vi "GenCMSMismatchFile.vi"() -> ()   [LabVIEW 2016]
uses:
  CMSMismatch.ctl
  <vilib>/NI/GXML/GXML.lvlib
panel:
  in  "Save Path":path
  in  "CableMotorSensorMismatch":T1={"TotalCount"={"CableCount"=0, "MotorCount"=0, "SensorCount"=0}, "Matches"=[{"CableID"=4, "MotorID"=8, "SensorID"=8}, {"CableID"=1, "MotorID"=6, "SensorID"=8}, {"CableID"=2, "MotorID"=5, "SensorID"=5}, {"CableID"=3, "MotorID"=7, "SensorID"=4}, {"CableID"=4, "MotorID"=4, "SensorID"=2}]}
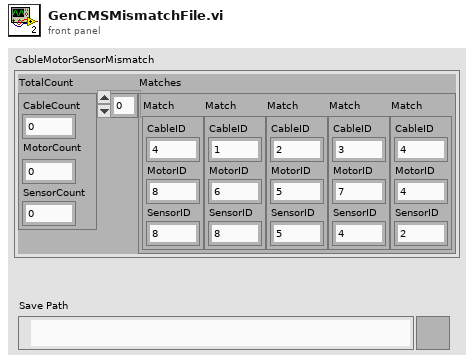
[diagram p1: front panel]
types:
  T1 = typedef "CMSMismatch.ctl" = cluster{"TotalCount":cluster{"CableCount":i32, "MotorCount":i32, "SensorCount":i32}, "Matches":cluster{"CableID":i32, "MotorID":i32, "SensorID":i32}[]}
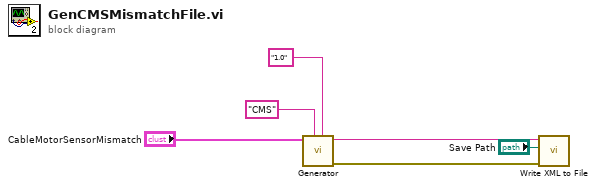
[diagram p0: block diagram]
diagram:
  n1 = call <vilib>:"Generator.vi"("Version String"="1.0", "Version Tag Name"="CMS", "Variant"="CableMotorSensorMismatch") -> ("error out"=w2:errorcluster, "XML String Out"=w3:string)  [unwired: 7 in]
  n2 = call <vilib>:"Write XML to File.vi"("error in"=w2, "XML File Path"="Save Path", "XML Input"=w3) -> ()  [unwired: 8 in, 1 out]
